vi "MagX Events to Listbox.vi"(8 "error in":errorcluster, 10 "Experiments":T1[](array[typedef]), 11 "Listbox ref":refnum<vi>) -> (0 "error out":errorcluster, 3 "Listbox ref out":refnum<vi>)   [LabVIEW 2024]
uses:
  Experiment info.ctl
panel:
  out "Listbox out":i32(listbox)
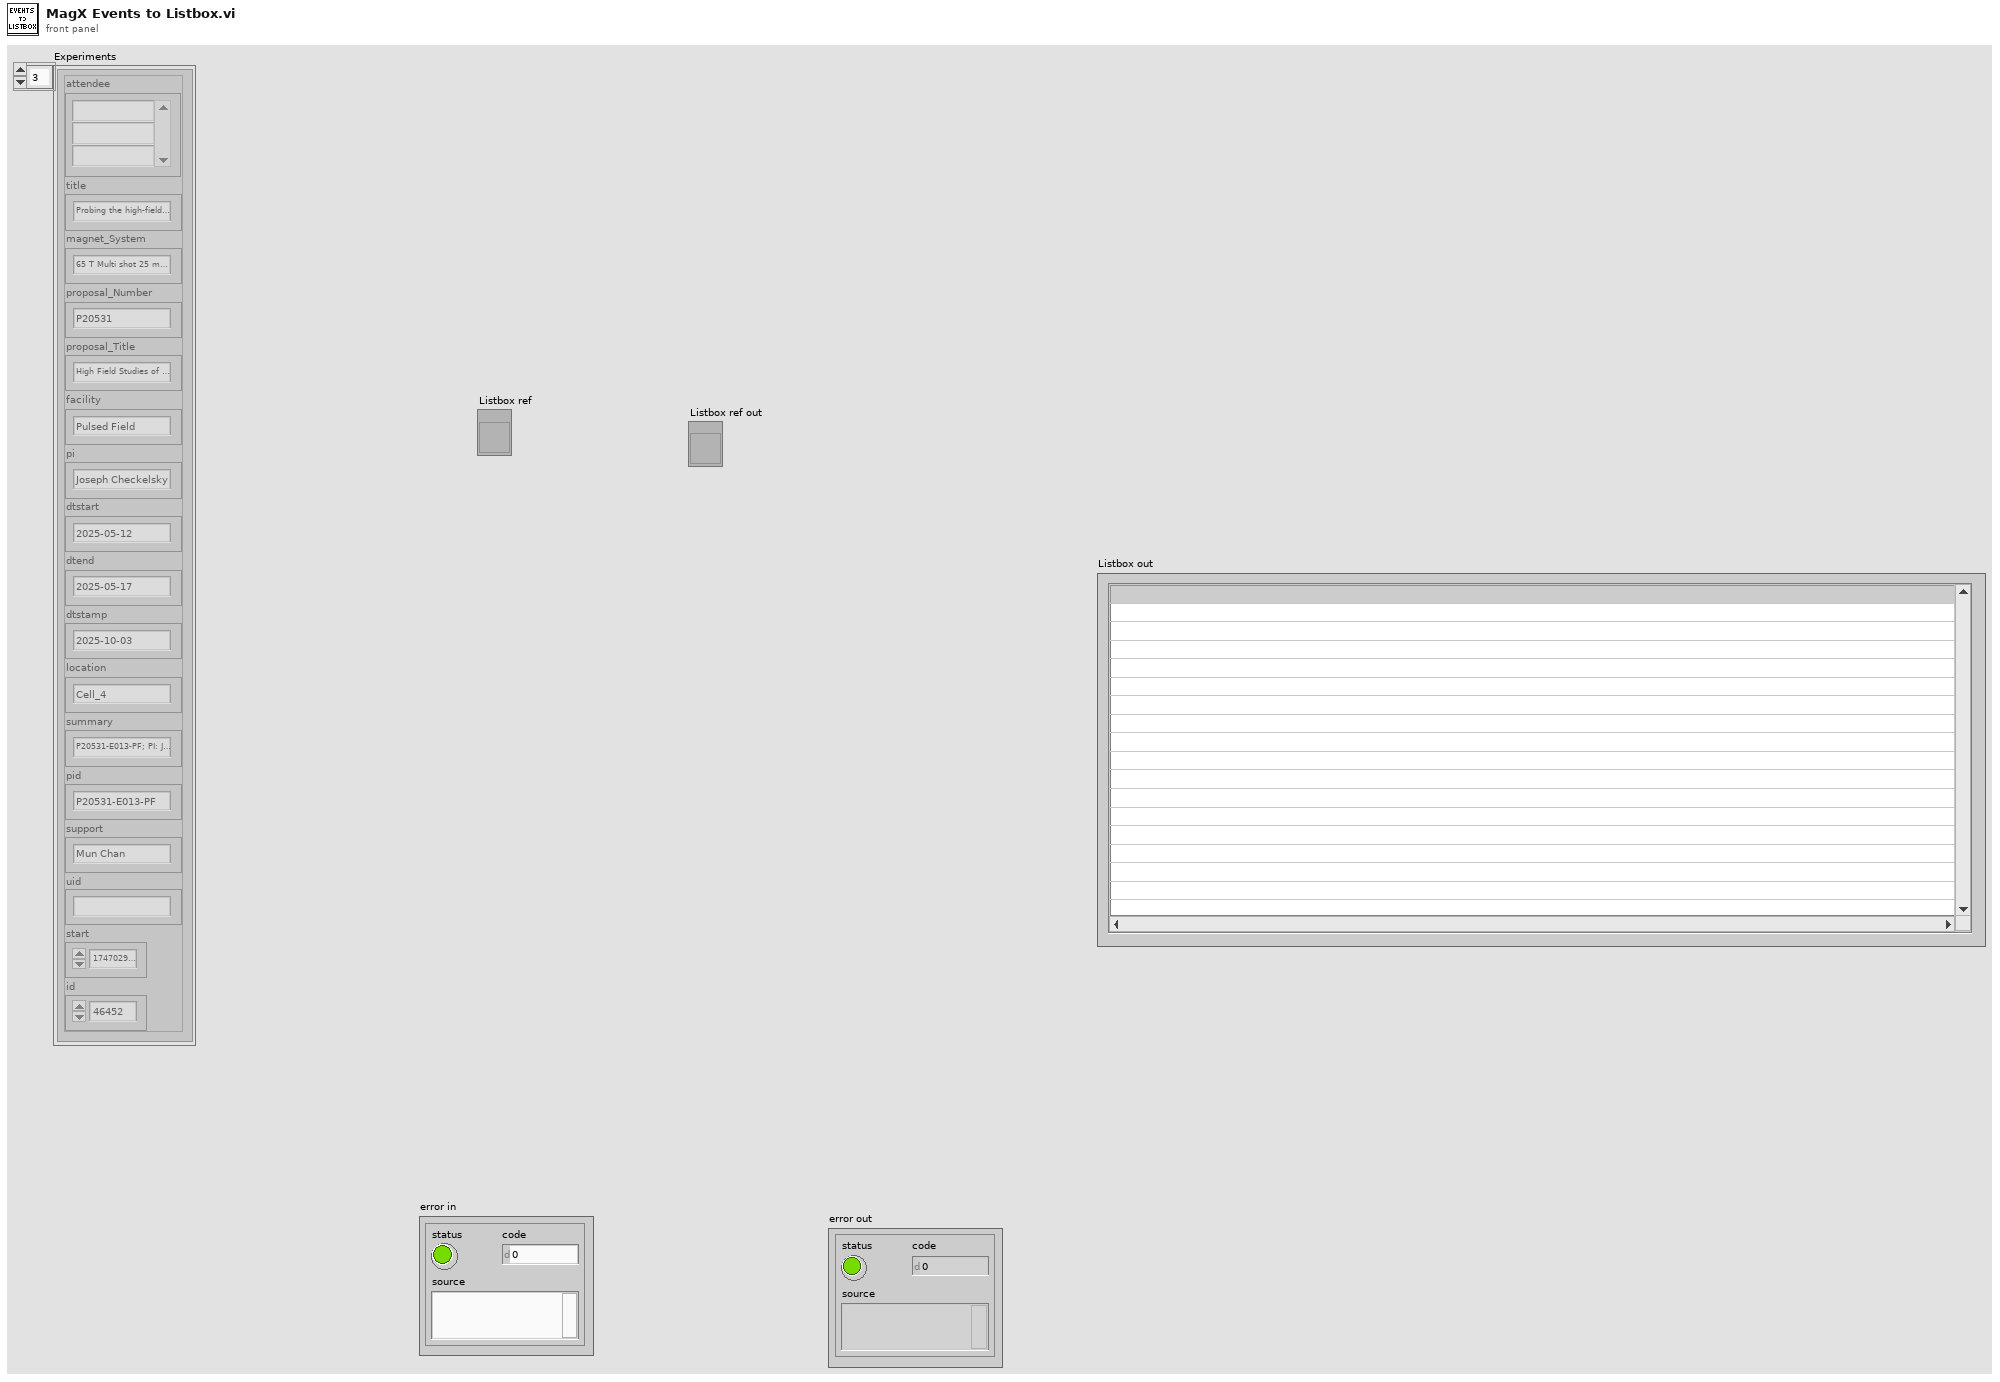
[diagram p1: front panel]
types:
  T1 = typedef "Experiment info.ctl" = cluster{"attendee":string[], "title":string, "magnet_System":string, "proposal_Number":string, "proposal_Title":string, "facility":string, "pi":string, "dtstart":string, "dtend":string, "dtstamp":string, "location":string, "summary":string, "pid":string, "support":string, "uid":string, "start":u64, "id":u64}
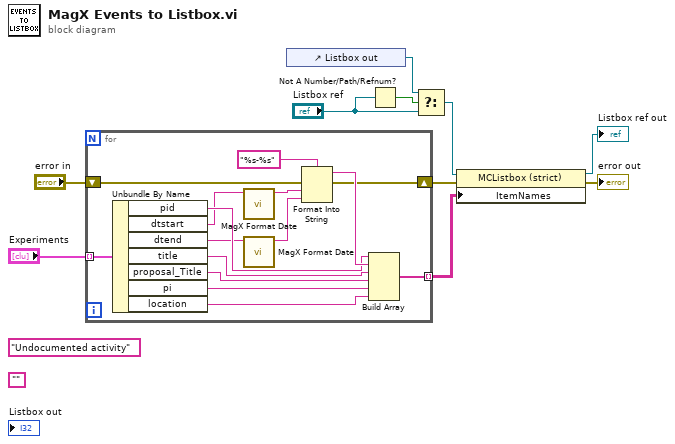
[diagram p0: block diagram]
diagram:
  (unwired) ""
  (unwired) "Undocumented activity"
  n1 = for {
    shift-right: [w23] -> w7
    shift-left: "error in" -> [w11]
    tunnel: [w22] -> w6 mode=indexing
    tunnel: "Experiments" -> [w21] mode=indexing
    n2 = Unbundle By Name(w21) -> ("pid"=w20:string, "dtstart"=w16:string, "dtend"=w14:string, "title"=w19:string, "proposal_Title"=w18:string, "pi"=w17:string, "location"=w12:string)
    n3 = call "MagX Format Date.vi"("String"=w16) -> ("String out"=w15:string)  [unwired: 8 in, 2 out]
    n4 = call "MagX Format Date.vi"("String"=w14) -> ("String out"=w13:string)  [unwired: 8 in, 2 out]
    n5 = Format Into String(format string="%s-%s", error in=w11, w15, w13) -> (resulting string=w24:string, error out=w23:errorcluster)  [unwired: 1 in]
    n6 = Build Array(w20, w24, w19, w18, w17, w12) -> (w22:string[])
  }
  n7 = control-ref of="Listbox out"() -> (w4:refnum<vi>)
  n8 = Not A Number/Path/Refnum?(number/path/refnum="Listbox ref") -> (NaN/Path/Refnum?=w5:bool)
  n9 = Select(t=w4, s=w5, f="Listbox ref") -> (s? t:f=w2:refnum<vi>)
  n10 = property class="MCListbox (strict)"(reference=w2, error in=w7, "ItemNames"=w6) -> (reference out=→"Listbox ref out":refnum<vi>, error out=→"error out":errorcluster)
